vi "Fuji Delta Single Motor Test.vi"() -> ()   [LabVIEW 2014]
uses:
  ALPHA5 RS485/typedefs/Port Selection Info.ctl
  Delta Robot/Fuji Delta Robot.lvclass/Fuji Delta Robot.ctl
  ALPHA5 RS485/Classes/FujiMotor/FujiMotor.lvclass
  Delta Robot/Fuji Delta Robot.lvclass
  ALPHA5 RS485/ALPHA5 RS485.lvlib
panel:
  out "Waveform Chart":cluster{"Slide":dbl, "ENC Pos":i32}(graph)
  in  "Inst Vel":i32=5000
  in  "ON/OFF":bool
  in  "stop":bool
  in  "Slide":dbl(slide) scale=-10000.0..10000.0
  in  "Port Selection Info In":T1={"Port Name"="COM5", "Amplifier Num"=1, "Baud Rate"=38400, "Char Formation"=enum."0"} {"Baud Rate" items=["38400"=38400, "19200"=19200, "9600"=9600, "115200"=0]; "Amplifier Num" max=31}
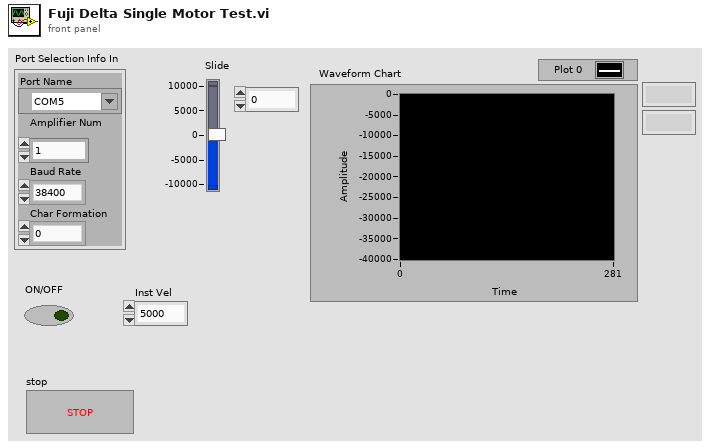
[diagram p1: front panel]
types:
  T1 = typedef "ALPHA5 RS485.lvlib/Port Selection Info.ctl" = cluster{"Port Name":refnum<visa-resource-name>, "Amplifier Num":u8, "Baud Rate":u32, "Char Formation":enum16{"0", "1", "2", "3", "4", "5"}}
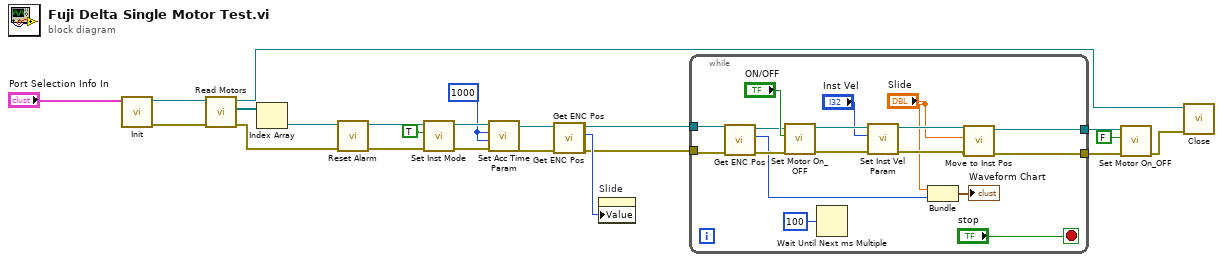
[diagram p0: block diagram]
diagram:
  w15 = 1000 ("ACC Time")
  n1 = call "Init.vi"("Port Selection Info In"="Port Selection Info In") -> ("error out"=w20:errorcluster, "Fuji Delta out"=w21:refnum<class "Fuji Delta Robot.lvclass">)  [unwired: 9 in]
  n2 = call "Read Motors.vi"("error in (no error)"=w20, "Fuji Delta Robot in"=w21) -> ("error out"=w1:errorcluster, "Motors"=w19:refnum<class "FujiMotor.lvclass">[], "Fuji Delta Robot out"=w13:refnum<class "Fuji Delta Robot.lvclass">)  [unwired: 7 in]
  n3 = Index Array(array=w19) -> (element=w2:refnum<class "FujiMotor.lvclass">)  [unwired: 1 in]
  n4 = call "Reset Alarm.vi"("error in (no error)"=w1, "FujiMotor in"=w2) -> ("error out"=w3:errorcluster, "FujiMotor out"=w4:refnum<class "FujiMotor.lvclass">)  [unwired: 8 in]
  n5 = call "Set Inst Mode.vi"("error in (no error)"=w3, "ABS/INC"=TRUE, "FujiMotor in"=w4) -> ("error out"=w16:errorcluster, "FujiMotor out"=w17:refnum<class "FujiMotor.lvclass">)  [unwired: 7 in]
  n6 = call "Set Acc Time Param.vi"("error in (no error)"=w16, "DEC Time"=w15, "ACC Time"=w15, "FujiMotor in"=w17) -> ("error out"=w6:errorcluster, "FujiMotor out"=w8:refnum<class "FujiMotor.lvclass">)  [unwired: 6 in]
  n7 = call "Get ENC Pos.vi"("FujiMotor in"=w8) -> ("ENC Pos"=w14:i32)  [unwired: 8 in, 2 out]
  n8 = call "Get ENC Pos.vi"("error in (no error)"=w6, "FujiMotor in"=w8) -> ("error out"=w5:errorcluster, "FujiMotor out"=w7:refnum<class "FujiMotor.lvclass">)  [unwired: 7 in, 1 out]
  n9 = property on="Slide" class="Slide (strict)"("Value"=w14) -> ()  [unwired: 2 in, 2 out]
  n10 = while {
    tunnel: w7 -> [w30]
    tunnel: w5 -> [w29]
    tunnel: [w32] -> w11
    tunnel: [w31] -> w12
    stop <- "stop" stop-if-true
    n11 = call "Get ENC Pos.vi"("error in (no error)"=w29, "FujiMotor in"=w30) -> ("error out"=w28:errorcluster, "ENC Pos"=w25:i32, "FujiMotor out"=w27:refnum<class "FujiMotor.lvclass">)  [unwired: 7 in]
    n12 = call "Set Motor On_OFF.vi"("error in (no error)"=w28, "ON/OFF"="ON/OFF", "FujiMotor in"=w27) -> ("error out"=w37:errorcluster, "FujiMotor out"=w36:refnum<class "FujiMotor.lvclass">)  [unwired: 7 in]
    n13 = Wait Until Next ms Multiple(millisecond multiple=u32 100) -> ()  [unwired: 1 out]
    n14 = call "Set Inst Vel Param.vi"("error in (no error)"=w37, "Inst Vel"="Inst Vel", "FujiMotor in"=w36) -> ("error out"=w33:errorcluster, "FujiMotor out"=w34:refnum<class "FujiMotor.lvclass">)  [unwired: 7 in]
    n15 = Bundle("Slide"="Slide", "ENC Pos"=w25) -> (→"Waveform Chart":cluster{"Slide":dbl, "ENC Pos":i32})  [unwired: 1 in]
    n16 = call "Move to Inst Pos.vi"("error in (no error)"=w33, "Inst Pos"="Slide", "FujiMotor in"=w34) -> ("error out"=w32:errorcluster, "FujiMotor out"=w31:refnum<class "FujiMotor.lvclass">)  [unwired: 7 in]
  }
  n17 = call "Set Motor On_OFF.vi"("error in (no error)"=w11, "ON/OFF"=FALSE, "FujiMotor in"=w12) -> ("error out"=w10:errorcluster)  [unwired: 7 in, 1 out]
  n18 = call "Close.vi"("error in (no error)"=w10, "Fuji Delta in"=w13) -> ()  [unwired: 9 in, 1 out]
